vi "_CSMObj-Message Check.vi"(6 "CSM":string, 8 "Error In":errorcluster caption="error in (no error)", 10 "Message":string, 11 "CSMQ In":T1={"info"={"Module Name"="", "Requested Name"="", "Group Name"="", "Mode"=enum."Stand Alone", "Allowed Messages"=[]}, "Refs"={"WatchDogQ"=refnum, "CSMDataDVR"=refnum, "Queue"={"HPriorityQ"=refnum, "LowPriorityQ"=refnum}, "GroupDataDVR"=refnum, "TagMap"=refnum, "ExitEvent"=refnum, "NewStateEvent"=refnum, "StatusEvent"=refnum, "InterruptEvent"=refnum}}) -> (0 "error out":errorcluster, 2 "Message (Dup)":string, 3 "CSMQ Out":T1={"info"={"Module Name"="", "Requested Name"="", "Group Name"="", "Mode"=enum."Stand Alone", "Allowed Messages"=[]}, "Refs"={"WatchDogQ"=refnum, "CSMDataDVR"=refnum, "Queue"={"HPriorityQ"=refnum, "LowPriorityQ"=refnum}, "GroupDataDVR"=refnum, "TagMap"=refnum, "ExitEvent"=refnum, "NewStateEvent"=refnum, "StatusEvent"=refnum, "InterruptEvent"=refnum}})   [LabVIEW 2017, in "Communicable State Machine.lvlib"]
uses:
  Communicable State Machine.lvlib
  _CSMObj.ctl
  _CSMObj-Info.ctl
  Typedef/_CSM_MODE.ctl
  _CSMObj-Refs.ctl
  _CSMObj-Data.ctl
  Priority Queue/Priority Queue.ctl
  Typedef/_Cross CSM State Data.ctl
  Typedef/_CSM_MSG_TYPE.ctl
  Typedef/_Cross CSM State Response.ctl
  Typedef/_CSM_Response Source Message.ctl
  Priority Queue/def-Data(LowPRI-Q).ctl
  _CSMObj-ModeData.ctl
  Typedef/_CSM Status Change Event Data.ctl
  _Shared/CSM Shared.lvlib
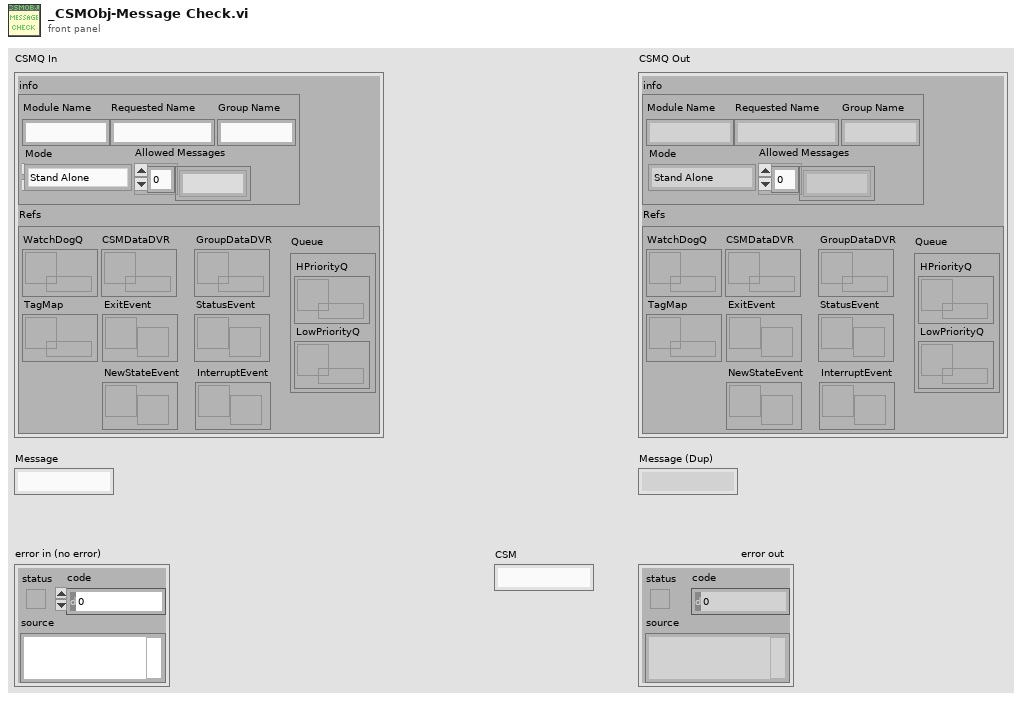
[diagram p1: front panel]
types:
  T1 = typedef "Communicable State Machine.lvlib/_CSMObj.ctl" = cluster{"info":T2, "Refs":T4}
  T2 = typedef "Communicable State Machine.lvlib/_CSMObj-Info.ctl" = cluster{"Module Name":string, "Requested Name":string, "Group Name":string, "Mode":T3, "Allowed Messages":string[]}
  T3 = typedef "Communicable State Machine.lvlib/_CSM_MODE.ctl" = enum16{"Not Exist", "Stand Alone", "CSM", "Worker", "Worker Agent", "Chain Node", "Chain"}
  T4 = typedef "Communicable State Machine.lvlib/_CSMObj-Refs.ctl" = cluster{"WatchDogQ":refnum<queue>, "CSMDataDVR":refnum<data-value>, "Queue":T5, "GroupDataDVR":refnum<data-value>, "TagMap":refnum<data-value>, "ExitEvent":refnum<user-event>, "NewStateEvent":refnum<user-event>, "StatusEvent":refnum<user-event>, "InterruptEvent":refnum<user-event>}
  T5 = typedef "Communicable State Machine.lvlib/Priority Queue.ctl" = cluster{"HPriorityQ":refnum<queue>, "LowPriorityQ":refnum<queue>}
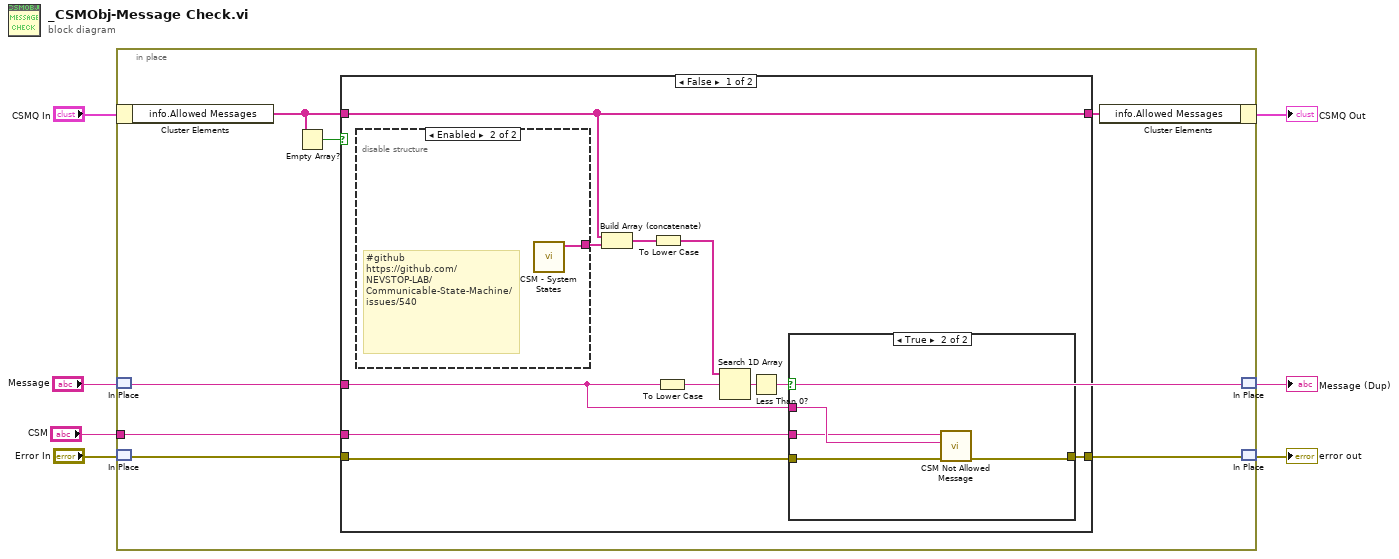
[diagram p0: block diagram]
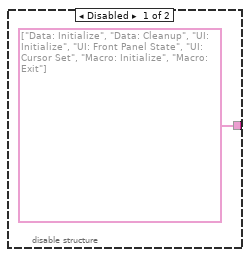
[diagram p2: hidden frame]
diagram:
  n1 = in-place "In Place Element Structure" {
    in-place-border: "CSM" -> [w8]
    n2 = in-place-cluster #1("CSMQ In") -> ("info.Allowed Messages"=w13:string[])
    n3 = in-place-match #2("Message") -> (w14:string)
    n4 = in-place-match #3("Error In") -> (w9:errorcluster)
    n5 = Empty Array?(array=w13) -> (empty?=w12:bool)
    n6 = case shown="False" w12 {
      tunnel: w14 -> [w24 _]
      tunnel: w13 -> [w19 w34]
      tunnel: [w19 w34] -> w11
      tunnel: [w22 w33] -> w10
      tunnel: w9 -> [w21 w33]
      tunnel: w8 -> [w17 _]
      frame False {
        n7 = disable-structure shown="Enabled" {
          disable-tunnel: [string[] ["Data: Initialize", "Data: Cleanup", "UI: Initialize", "UI: Front Panel State", "UI: Cursor Set", "Macro: Initialize", "Macro: Exit"] ("array") w27] -> w16
          frame Disabled {
          }
          frame Enabled {
            # "#github\nhttps://github.com/NEVSTOP-LAB/Communicable-State-Machine/issues/540"
            n8 = call "CSM - System States.vi"() -> ("items to filter"=w27:string[])  [unwired: 11 in]
          }
        }
        n9 = Build Array (concatenate)(w19, w16) -> (w18:string[])
        n10 = To Lower Case(string=w18) -> (all lower case string=w15:string[])
        n11 = To Lower Case(string=w24) -> (all lower case string=w20:string)
        n12 = Search 1D Array(1D array=w15, element=w20) -> (index of element=w25:i32)  [unwired: 1 in]
        n13 = Less Than 0?(x=w25) -> (x < 0?=w23:bool)
        n14 = case shown="True" w23 {
          tunnel: w24 -> [_ w31]
          tunnel: [w28 w30] -> w22
          tunnel: w21 -> [w28 w32]
          tunnel: w17 -> [_ w29]
          frame False {
          }
          frame True {
            n15 = call "CSM Not Allowed Message.vi"("error in (no error)"=w32, "State"=w31, "CSM"=w29) -> ("error out"=w30:errorcluster)  [unwired: 8 in]
          }
        }
      }
      frame True {
      }
    }
    n16 = in-place-cluster #1("info.Allowed Messages"=w11) -> (→"CSMQ Out":T1)
    n17 = in-place-match #2(w14) -> (→"Message (Dup)":string)
    n18 = in-place-match #3(w10) -> (→"error out":errorcluster)
  }
